vi "CreateSimulatedData.vi"(11 "data in":sgl[][](array[numeric])) -> (3 "data out":sgl[][](array[numeric]))   [LabVIEW 2017, in "IrAcquisition.lvlib"]
uses:
  <vilib>/addons/InsightCM/Devices/Shared/Ir/IrAcquisition/IrAcquisition.lvlib
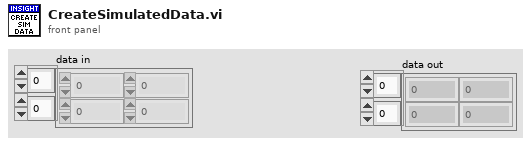
[diagram p1: front panel]
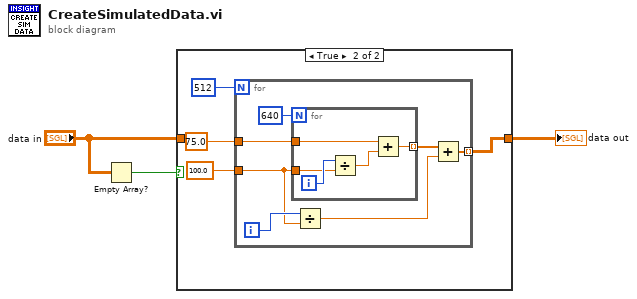
[diagram p0: block diagram]
diagram:
  n1 = Empty Array?(array="data in") -> (empty?=w3:bool)
  n2 = case shown="True" w3 {
    tunnel: [w4 w5] -> w2
    tunnel: "data in" -> [w4 _]
    frame False {
    }
    frame True {
      n3 = for {
        N: 512 -> [_]
        tunnel: sgl 100.0 -> [w13]
        tunnel: sgl 75.0 -> [w12]
        tunnel: [w9] -> w5 mode=indexing
        i -> [w14]
        n4 = for {
          N: 640 -> [_]
          tunnel: w13 -> [w19]
          tunnel: w12 -> [w17]
          tunnel: [w16] -> w11 mode=indexing
          i -> [w20]
          n5 = Divide(x=w20, y=w19) -> (x/y=w18:sgl)
          n6 = Add(x=w17, y=w18) -> (x+y=w16:sgl)
        }
        n7 = Divide(x=w14, y=w13) -> (x/y=w10:sgl)
        n8 = Add(x=w11, y=w10) -> (x+y=w9:sgl[])
      }
    }
  }
  "data out" <- w2
